vi "Set Sart Cameras.vi"(8 "error in (no error)":errorcluster, 9 "Camera 3":T1="dummy", 10 "Camera 2":T1="dummy", 11 "HIJ 4 Aligment Cams Launcher in":refnum<class "HIJ 3 Aligment Cams Launcher.lvclass">) -> (0 "error out":errorcluster, 3 "HIJ 4 Aligment Cams Launcher out":refnum<class "HIJ 3 Aligment Cams Launcher.lvclass">)   [LabVIEW 2014, in "HIJ 3 Alignment Cams App.lvlib" / "HIJ 3 Aligment Cams Launcher.lvclass"]
uses:
  HIJ 3 Aligment Cams Launcher.lvclass
  <vilib>/userdefined/High Color/IMAQdx.ctl
  HIJ 3 Alignment Cams App/HIJ 3 Alignment Cams App.lvclass
  HIJ Vision Launcher/HIJ Vision Launcher/HIJ Vision Launcher.lvclass/HIJ Vision Launcher.ctl
  HIJ 3 Alignment Cams App/HIJ 3 Alignment Cams App.lvclass/HIJ 3 Alignment Cams App.ctl
  HIJ Vision Launcher/HIJ Vision Launcher/Read HIJ Vision Camera App.vi
  HIJ 3 Alignment Cams App/Write Start Camera 2.vi
  HIJ 3 Alignment Cams App/Write Start Camera 3.vi
  HIJ Vision Launcher/HIJ Vision Launcher/Write HIJ Vision Camera App.vi
  Viewable Actor/ViewableActor/ViewableActor.lvclass
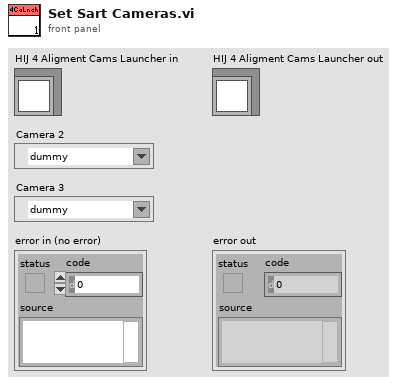
[diagram p1: front panel]
types:
  T1 = typedef "IMAQdx.ctl" = refnum<k21>
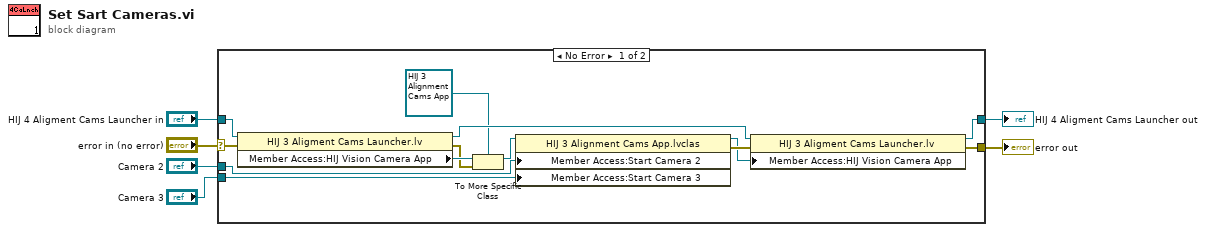
[diagram p0: block diagram]
diagram:
  n1 = case shown="No Error" "error in (no error)" {
    selector: "error in (no error)" -> [w9 w21]
    tunnel: [w8 w21] -> w5
    tunnel: [w17 w20] -> w3
    tunnel: "HIJ 4 Aligment Cams Launcher in" -> [w19 w20]
    tunnel: "Camera 2" -> [w12 _]
    tunnel: "Camera 3" -> [w11 _]
    frame No Error {
      n2 = property class="HIJ 3 Aligment Cams Launcher.lv"(reference=w19, error in=w9) -> (reference out=w18:refnum<class "HIJ 3 Aligment Cams Launcher.lvclass">, error out=w13:errorcluster, "Member Access:HIJ Vision Camera App"=w16:refnum<class "ViewableActor.lvclass">)
      n3 = To More Specific Class(target class=refnum<class "HIJ 3 Alignment Cams App.lvclass"> refnum ("HIJ 4 Alignment Cams App.lvlib:HIJ 4 Alignment Cams App.lvclass"), reference=w16, error in=w13) -> (specific class reference=w15:refnum<class "HIJ 3 Alignment Cams App.lvclass">)  [unwired: 1 out]
      n4 = property class="HIJ 3 Alignment Cams App.lvclas"(reference=w15, "Member Access:Start Camera 2"=w12, "Member Access:Start Camera 3"=w11) -> (reference out=w7:refnum<class "HIJ 3 Alignment Cams App.lvclass">, error out=w10:errorcluster)  [unwired: 1 in]
      n5 = property class="HIJ 3 Aligment Cams Launcher.lv"(reference=w18, error in=w10, "Member Access:HIJ Vision Camera App"=w7) -> (reference out=w17:refnum<class "HIJ 3 Aligment Cams Launcher.lvclass">, error out=w8:errorcluster)
    }
    frame Error {
    }
  }
  "error out" <- w5
  "HIJ 4 Aligment Cams Launcher out" <- w3
